vi "Empty Scrollback.vi"(8 "error in (no error)":errorcluster, 11 "TermBuffer in":refnum<class "TermBuffer.lvclass">) -> (0 "error out":errorcluster, 3 "TermBuffer out":refnum<class "TermBuffer.lvclass">)   [LabVIEW 2020, in "Terminal.lvlib" / "TermBuffer.lvclass"]
uses:
  TermBuffer.lvclass
  TermBuffer.lvclass/TermBuffer.ctl
  TermLine/TermLine.lvclass
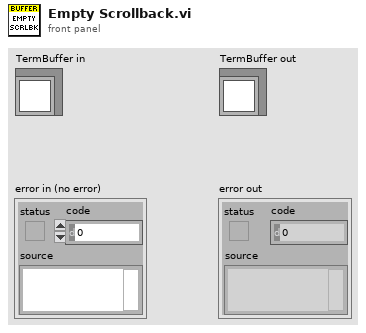
[diagram p1: front panel]
types:
  T1 = typedef "Terminal.lvlib/TermBuffer.lvclass/Ref Data.ctl" = cluster{"Lines":refnum<class "TermLine.lvclass">[], "Rows":i32, "Cols":i32}
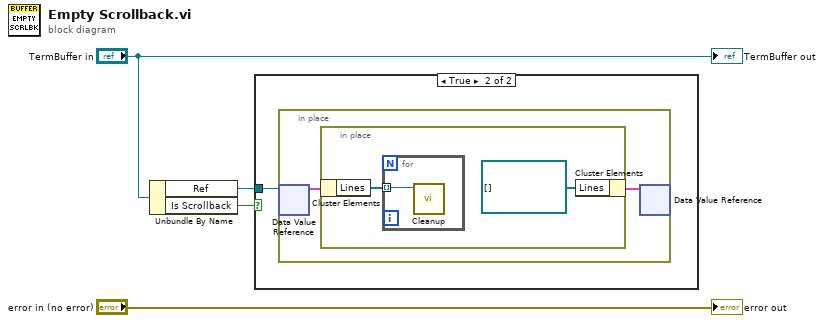
[diagram p0: block diagram]
diagram:
  n1 = Unbundle By Name("TermBuffer in") -> ("Ref"=w3:refnum<data-value>, "Is Scrollback"=w1:bool)
  n2 = case shown="True" w1 {
    tunnel: w3 -> [_ w5]
    frame False {
    }
    frame True {
      n3 = in-place {
        n4 = in-place-dvr #1(w5) -> (w7:T1)  [unwired: 1 out]
        n5 = in-place {
          n6 = in-place-cluster #2(w7) -> ("Lines"=w8:refnum<class "TermLine.lvclass">[])
          n7 = for {
            tunnel: w8 -> [w10] mode=indexing
            n8 = call "Cleanup.vi"("TermLine in"=w10) -> ()  [unwired: 10 in, 1 out]
          }
          n9 = in-place-cluster #2("Lines"=refnum<class "TermLine.lvclass">[] []) -> (w6:T1)
        }
        n10 = in-place-dvr #1(w6) -> ()  [unwired: 2 out]
      }
    }
  }
  "error out" <- "error in (no error)"
  "TermBuffer out" <- "TermBuffer in"
